vi "StopMods.vi"(8 "ErrorArray In":errorcluster[](array[cluster]), 11 "Test.lvclass":refnum<class "Test.lvclass">) -> (0 "ErrorArray Out":errorcluster[](array[cluster]), 3 "Test.lvclass":refnum<class "Test.lvclass">)   [LabVIEW 2018, in "Test.lvclass"]
doc: "Stops all modules based on the Test Class information (Clone Registration, Module ID, and Module list)."
uses:
  Test.lvclass
  Test.lvclass/Test.ctl
  <userlib>/NIST/ModuleAdminLib/CloneRegistration/CloneRegistration.lvclass
  Accessors/Write ModuleIDs.vi
  Accessors/Write ModuleList.vi
  Accessors/Write CloneReg.vi
  Accessors/Read CloneReg.vi
  Accessors/Read ModuleIDs.vi
  Accessors/Read ModuleList.vi
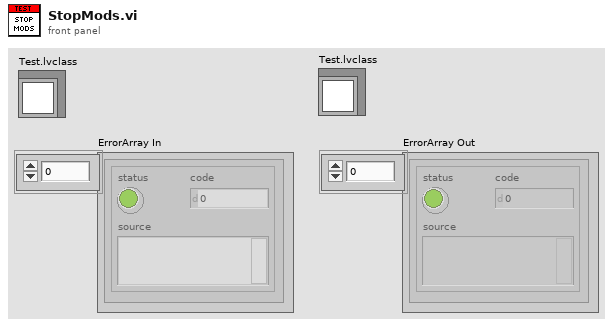
[diagram p1: front panel]
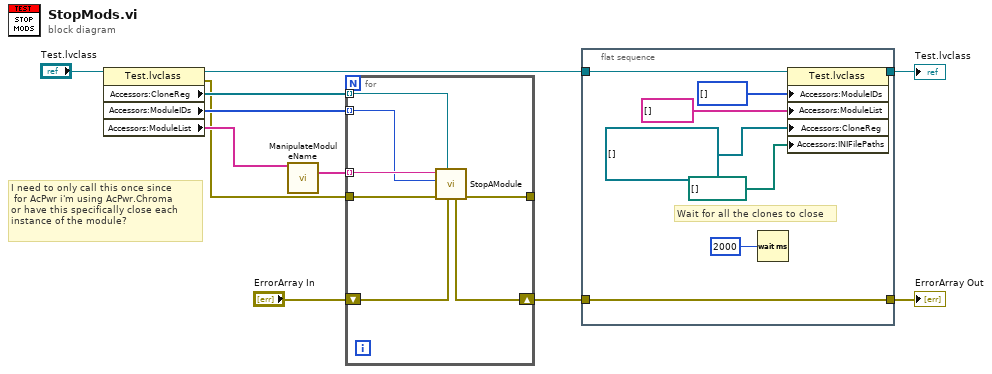
[diagram p0: block diagram]
diagram:
  # "I need to only call this once since\n for AcPwr i'm using AcPwr.Chroma\nor have this specifically close each \ninstance of the module?"
  n1 = property class="Test.lvclass"(reference="Test.lvclass") -> (reference out=w9:refnum<class "Test.lvclass">, error out=w6:errorcluster, "Accessors:CloneReg"=w10:refnum<data-value>[], "Accessors:ModuleIDs"=w8:i32[], "Accessors:ModuleList"=w7:string[])  [unwired: 1 in]
  n2 = call "ManipulateModuleName.vi"("ModuleListArrayIn"=w7) -> ("BeforeMatch:ModuleListArray"=w1:string[])  [unwired: 9 in, 5 out]
  n3 = for {
    shift-right: [w15] -> w2
    shift-left: "ErrorArray In" -> [w16]
    tunnel: w10 -> [w14] mode=indexing
    tunnel: w8 -> [w13] mode=indexing
    tunnel: w1 -> [w17] mode=indexing
    tunnel: w6 -> [w12]
    tunnel: [w12] -> _
    n4 = call "StopAModule.vi"("ErrorArray In"=w16, "Module Clone Reg"=w14, "error in (no error)"=w12, "Module ID"=w13, "Module Name (e.g. Sensor, Digitizer, etc.)"=w17) -> ("ErrorArray Out"=w15:errorcluster[])  [unwired: 6 in]
  }
  n5 = flat-sequence {
    tunnel: w9 -> [w25]
    tunnel: [w24] -> w4
    tunnel: [w19] -> w3
    tunnel: w2 -> [w19]
    frame #0 {
      # "Wait for all the clones to close"
      n6 = Wait (ms)(milliseconds to wait=u32 2000) -> ()  [unwired: 1 out]
      n7 = property class="Test.lvclass"(reference=w25, "Accessors:ModuleIDs"=i32[] [] ("ModuleIDs"), "Accessors:ModuleList"=string[] [] ("ModuleList"), "Accessors:CloneReg"=refnum<data-value>[] [] ("CloneReg"), "Accessors:INIFilePaths"=path[] [] ("INIFilePaths")) -> (reference out=w24:refnum<class "Test.lvclass">)  [unwired: 1 in, 1 out]
    }
  }
  "Test.lvclass" <- w4
  "ErrorArray Out" <- w3
